vi "Lab 2 Q4.vi"() -> ()   [LabVIEW 2016]
panel:
  out "String":string
  in  "Stop":bool
  in  "X":bool
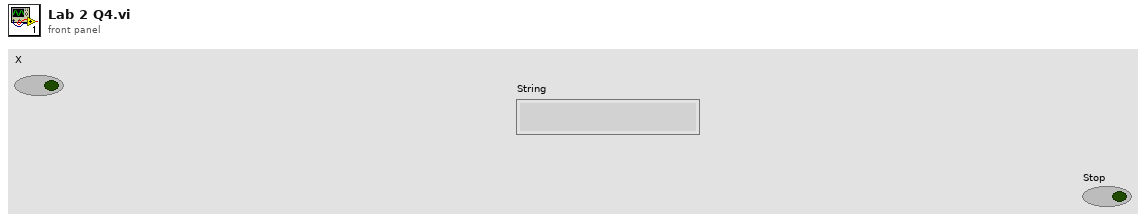
[diagram p1: front panel]
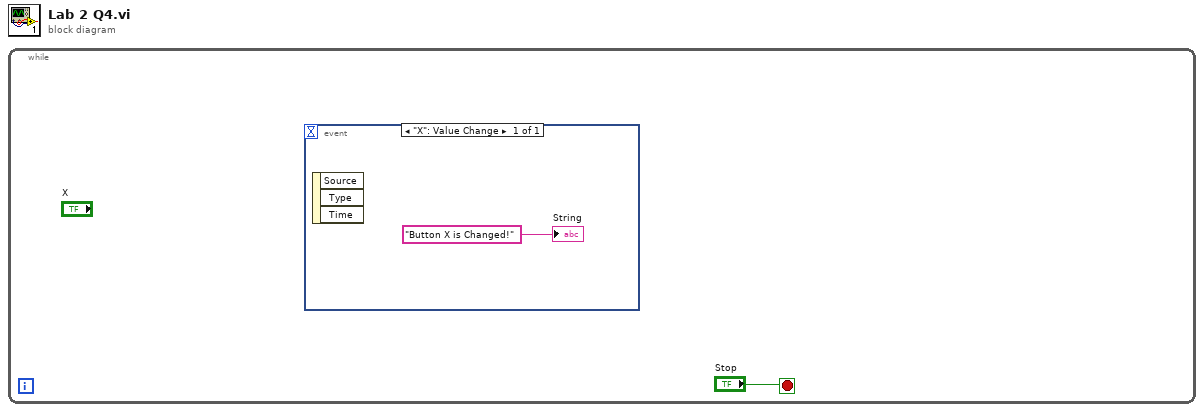
[diagram p0: block diagram]
diagram:
  n1 = while {
    stop <- "Stop" stop-if-true
    n2 = event shown="[0] \"X\": Value Change" {
      selector: _ -> [_]
      dyn-events: _ -> [_]
      timeout: _ -> [_]
      event "X": Value Change {
        n3 = event-data() -> ()  [unwired: 1 in, 3 out]
        "String" <- "Button X is Changed!"
      }
    }
  }
